vi "displayConfigurableElements.vi"(11 "ConfigurationThisComponent in":refnum<class "ConfigurationTestParameters.lvclass">) -> (3 "ConfigurationThisComponent out":refnum<class "ConfigurationTestParameters.lvclass">)   [LabVIEW 2016, in "ConfigurationTestParameters.lvclass"]
uses:
  ConfigurationTestParameters.lvclass
  Common_Log/Config/Log.ctl
  Typedefs/Device Configuration Tests.ctl
  Typedefs/1-Wire Test.ctl
  Typedefs/Collection Settings.ctl
  Typedefs/TestExecutionOrder.ctl
  Typedefs/TestScenarioTypes.ctl
  Typedefs/Set DAC Tests.ctl
  Typedefs/Set DAC Test.ctl
  Typedefs/Verify DAC Tests.ctl
  Typedefs/DAC Channels.ctl
  Typedefs/Verify DAC Test.ctl
  Typedefs/Verify Voltage Tests.ctl
  Typedefs/Verify Voltage Test.ctl
  Typedefs/Enable Disable.ctl
  Typedefs/Pressure Tests.ctl
  Typedefs/Pressure Test.ctl
  Common_Log/Log.lvlib
  Typedefs/ILCBTTypedefs.lvlib
panel:
  in  "ctrlRefArrayUsrEvnt":refnum<user-event>
  in  "ConfigTab":T1(tab)
  in  "TestDataLog":T2={"Log Directory"=path "", "Log Filename Base"="", "Max records per file"=1000, "Comment"=""} {"Max records per file" min=100 max=1000000}
  in  "TestExecutionOrder":T3
  in  "Collection Settings":T5={"Samples To Average"=1, "Test Delay"=0.01, "Linearity Step"=1024}
  in  "Device Configuration Tests":T6
  in  "Set DAC Tests":T8={"DAC = 0.00A"={"Command Value"=34224}, "DAC = 0.25A"={"Command Value"=42052}, "DAC = 0.5A"={"Command Value"=49879}, "DAC = 0.75A"={"Command Value"=57707}, "DAC = 1.0A"={"Command Value"=65535}, "DAC = -0.25A"={"Command Value"=26396}, "DAC = -0.5A"={"Command Value"=18568}, "DAC = -0.75A"={"Command Value"=10740}, "DAC = -1.0A"={"Command Value"=0}}
  in  "Verify DAC Tests":T10={"DAC A Channels"={"DAQ Channel 1 to Read"="ai5", "DAQ Channel 2 to Read"="ai6", "Resistor Ohms"=0.0}, "DAC B Channels"={"DAQ Channel 1 to Read"="ai7", "DAQ Channel 2 to Read"="ai8", "Resistor Ohms"=0.0}, "DAC = -1.00A"={"Expected Value"=-1.0, "Tolerance"=0.001}, "DAC = -0.75A"={"Expected Value"=-0.75, "Tolerance"=0.00075}, "DAC = -0.50A"={"Expected Value"=-0.5, "Tolerance"=0.0005}, "DAC = -0.25A"={"Expected Value"=-0.25, "Tolerance"=0.00025}, "DAC = 0.00A"={"Expected Value"=0.0, "Tolerance"=0.0001}, "DAC = 0.25A"={"Expected Value"=0.25, "Tolerance"=0.00025}, "DAC = 0.50A"={"Expected Value"=0.5, "Tolerance"=0.0005}, "DAC = 0.75A"={"Expected Value"=0.75, "Tolerance"=0.00075}, "DAC = 1.00A"={"Expected Value"=1.0, "Tolerance"=0.001}} {"DAC = 1.00A"."Tolerance" format="%.6f"; "DAC = 1.00A"."Expected Value" format="%.3f"; "DAC = 0.75A"."Tolerance" format="%.6f"; "DAC = 0.75A"."Expected Value" format="%.3f"; "DAC = 0.50A"."Tolerance" format="%.6f"; "DAC = 0.50A"."Expected Value" format="%.3f"; "DAC = 0.25A"."Tolerance" format="%.6f"; "DAC = 0.25A"."Expected Value" format="%.3f"; "DAC = 0.00A"."Tolerance" format="%.6f"; "DAC = 0.00A"."Expected Value" format="%.3f"; "DAC = -0.25A"."Tolerance" format="%.6f"; "DAC = -0.25A"."Expected Value" format="%.3f"; "DAC = -0.50A"."Tolerance" format="%.6f"; "DAC = -0.50A"."Expected Value" format="%.3f"; "DAC = -0.75A"."Tolerance" format="%.6f"; "DAC = -0.75A"."Expected Value" format="%.3f"; "DAC = -1.00A"."Tolerance" format="%.6f"; "DAC = -1.00A"."Expected Value" format="%.3f"; "DAC B Channels"."Resistor Ohms" format="%.3g"; "DAC A Channels"."Resistor Ohms" format="%.3g"}
  in  "Verify Voltage Tests":T13={"+3.3VD"={"DAQ Channel to Read"="ai0", "Expected Value"=3.3, "Tolerance"=0.0033}, "+5.1V"={"DAQ Channel to Read"="ai1", "Expected Value"=5.1, "Tolerance"=0.0051}, "RELVALV1"={"DAQ Channel to Read"="ai3", "Expected Value"=2.4, "Tolerance"=0.0024}, "RELVALV2"={"DAQ Channel to Read"="ai4", "Expected Value"=2.4, "Tolerance"=0.0024}} {"RELVALV2"."Tolerance" format="%.6f"; "RELVALV2"."Expected Value" format="%.3f"; "RELVALV1"."Tolerance" format="%.6f"; "RELVALV1"."Expected Value" format="%.3f"; "+5.1V"."Tolerance" format="%.6f"; "+5.1V"."Expected Value" format="%.3f"; "+3.3VD"."Tolerance" format="%.6f"; "+3.3VD"."Expected Value" format="%.3f"}
  in  "Enable Disable":T15={"Motor Enable"=1, "Motor Disable"=0, "Current Output Enable"=1, "Current Output Disable"=0, "Power Enable"=0, "Power Disable"=1, "Amplifier Enable"=0, "Amplifier Disable"=1}
  in  "Pressure Tests":T16={"0% Test"={"Command"=0, "Expected"=1933, "Tolerance"=492}, "25% Test"={"Command"=12322, "Expected"=4095, "Tolerance"=492}, "50% Test"={"Command"=26326, "Expected"=6553, "Tolerance"=492}, "75% Test"={"Command"=40329, "Expected"=9010, "Tolerance"=492}, "100% Test"={"Command"=54332, "Expected"=11468, "Tolerance"=492}, "Settling (ms)"=500, "Delay (ms)"=10}
  # "Unique ID Test"
  # "TEDS Status Test"
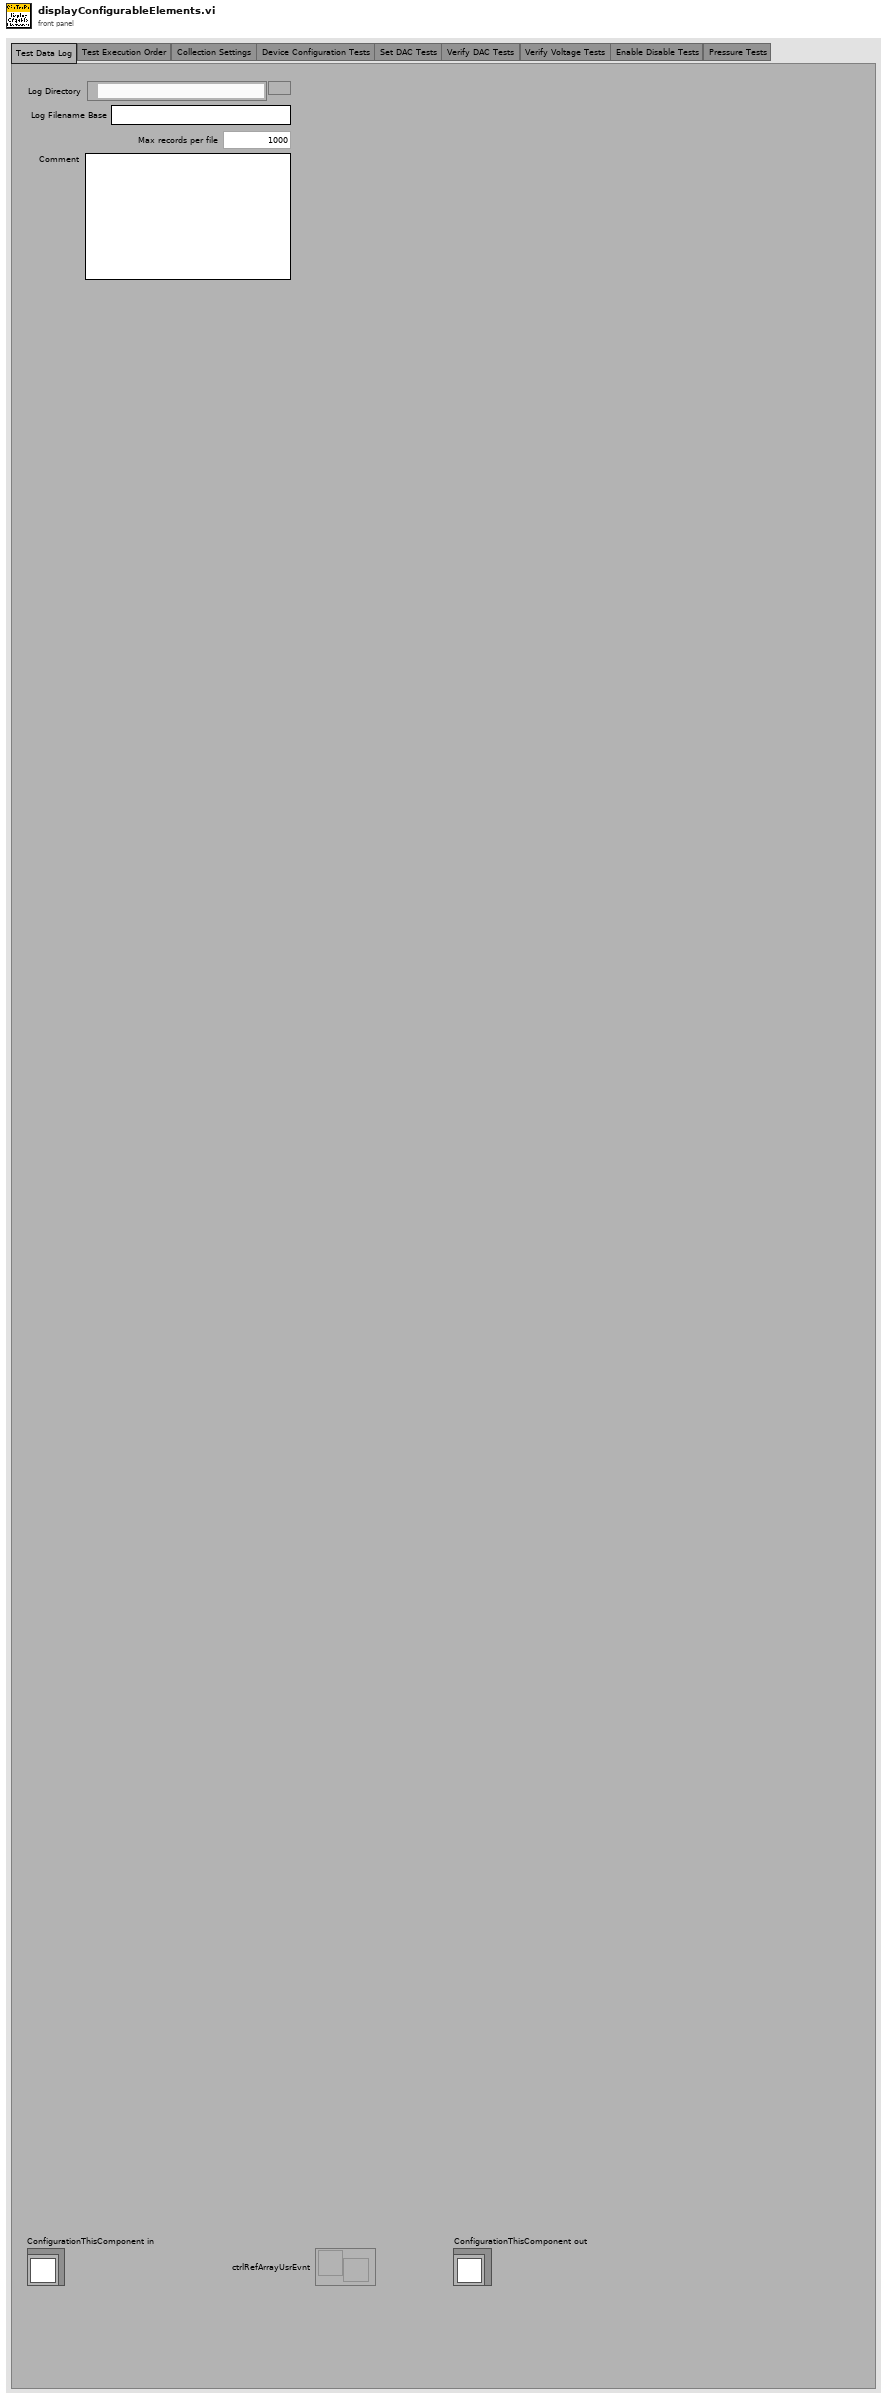
[diagram p1: front panel]
types:
  T1 = enum32{"Test Data Log", "Test Execution Order", "Collection Settings", "Device Configuration Tests", "Set DAC Tests", "Verify DAC Tests", "Verify Voltage Tests", "Enable Disable Tests", "Pressure Tests"}
  T2 = typedef "Log.lvlib/Log.ctl" = cluster{"Log Directory":path, "Log Filename Base":string, "Max records per file":u32, "Comment":string}
  T3 = typedef "ILCBTTypedefs.lvlib/TestExecutionOrder.ctl" = T4[]
  T4 = typedef "ILCBTTypedefs.lvlib/TestScenarioTypes.ctl" = enum16{"+3.3VD", "+5.1V", "+24V", "RELVALV1", "RELVALV2", "Verify DAC_A = -1.00A", "Verify DAC_A = -0.75A", "Verify DAC_A = -0.50A", "Verify DAC_A = -0.25A", "Verify DAC_A = 0.00A", "Verify DAC_A = 0.25A", "Verify DAC_A = 0.50A", "Verify DAC_A = 0.75A", "Verify DAC_A = 1.00A", "Verify DAC_B = -1.00A", "Verify DAC_B = -0.75A", "Verify DAC_B = -0.50A", "Verify DAC_B = -0.25A", "Verify DAC_B = 0.00A", "Verify DAC_B = 0.25A", "Verify DAC_B = 0.50A", "Verify DAC_B = 0.75A", "Verify DAC_B = 1.00A", "Set DAC_A = -1.00A", "Set DAC_A = -0.75A", "Set DAC_A = -0.50A", "Set DAC_A = -0.25A", "Set DAC_A = 0.00A", "Set DAC_A = 0.25A", "Set DAC_A = 0.50A", "Set DAC_A = 0.75A", "Set DAC_A = 1.00A", "Set DAC_B = -1.00A", "Set DAC_B = -0.75A", "Set DAC_B = -0.50A", "Set DAC_B = -0.25A", "Set DAC_B = 0.00A", "Set DAC_B = 0.25A", "Set DAC_B = 0.50A", "Set DAC_B = 0.75A", "Set DAC_B = 1.00A", "Set MTR_PWR = On", "Set MTR_PWR = Off", "Set OUTPUT = On", "Set OUTPUT = Off", "Verify OUTPUT = On", "Verify OUTPUT = Off", "Verify POWER = Ok", "Verify POWER = Fail", "Verify AMP1 = Ok", "Verify AMP1 = Fail", "Verify AMP2 = Ok", "Verify AMP2 = Fail", "P1 0%", "P1 25%", "P1 50%", "P1 75%", "P1 100%", "P2 0%", "P2 25%", "P2 50%", "P2 75%", "P2 100%", "P3 0%", "P3 25%", "P3 50%", "P3 75%", "P3 100%", "P4 0%", "P4 25%", "P4 50%", "P4 75%", "P4 100%", "DCA 1 Linearity", "DCA 2 Linearity"}
  T5 = typedef "ILCBTTypedefs.lvlib/Collection Settings.ctl" = cluster{"Samples To Average":i32, "Test Delay":dbl, "Linearity Step":i32}
  T6 = typedef "ILCBTTypedefs.lvlib/Device Configuration Tests.ctl" = cluster{"TEDS Status Test":T7, "Unique ID Length":u8}
  T7 = typedef "ILCBTTypedefs.lvlib/1-Wire Test.ctl" = cluster{"Expected Value":string}
  T8 = typedef "ILCBTTypedefs.lvlib/Set DAC Tests.ctl" = cluster{"DAC = 0.00A":T9, "DAC = 0.25A":T9, "DAC = 0.5A":T9, "DAC = 0.75A":T9, "DAC = 1.0A":T9, "DAC = -0.25A":T9, "DAC = -0.5A":T9, "DAC = -0.75A":T9, "DAC = -1.0A":T9}
  T9 = typedef "ILCBTTypedefs.lvlib/Set DAC Test.ctl" = cluster{"Command Value":u16}
  T10 = typedef "ILCBTTypedefs.lvlib/Verify DAC Tests.ctl" = cluster{"DAC A Channels":T11, "DAC B Channels":T11, "DAC = -1.00A":T12, "DAC = -0.75A":T12, "DAC = -0.50A":T12, "DAC = -0.25A":T12, "DAC = 0.00A":T12, "DAC = 0.25A":T12, "DAC = 0.50A":T12, "DAC = 0.75A":T12, "DAC = 1.00A":T12}
  T11 = typedef "ILCBTTypedefs.lvlib/DAC Channels.ctl" = cluster{"DAQ Channel 1 to Read":refnum<k21>, "DAQ Channel 2 to Read":refnum<k21>, "Resistor Ohms":dbl}
  T12 = typedef "ILCBTTypedefs.lvlib/Verify DAC Test.ctl" = cluster{"Expected Value":dbl, "Tolerance":dbl}
  T13 = typedef "ILCBTTypedefs.lvlib/Verify Voltage Tests.ctl" = cluster{"+3.3VD":T14, "+5.1V":T14, "RELVALV1":T14, "RELVALV2":T14}
  T14 = typedef "ILCBTTypedefs.lvlib/Verify Voltage Test.ctl" = cluster{"DAQ Channel to Read":refnum<k21>, "Expected Value":dbl, "Tolerance":dbl}
  T15 = typedef "ILCBTTypedefs.lvlib/Enable Disable.ctl" = cluster{"Motor Enable":u16, "Motor Disable":u16, "Current Output Enable":u16, "Current Output Disable":u16, "Power Enable":u16, "Power Disable":u16, "Amplifier Enable":u16, "Amplifier Disable":u16}
  T16 = typedef "ILCBTTypedefs.lvlib/Pressure Tests.ctl" = cluster{"0% Test":T17, "25% Test":T17, "50% Test":T17, "75% Test":T17, "100% Test":T17, "Settling (ms)":u16, "Delay (ms)":u16}
  T17 = typedef "ILCBTTypedefs.lvlib/Pressure Test.ctl" = cluster{"Command":u16, "Expected":u16, "Tolerance":u16}
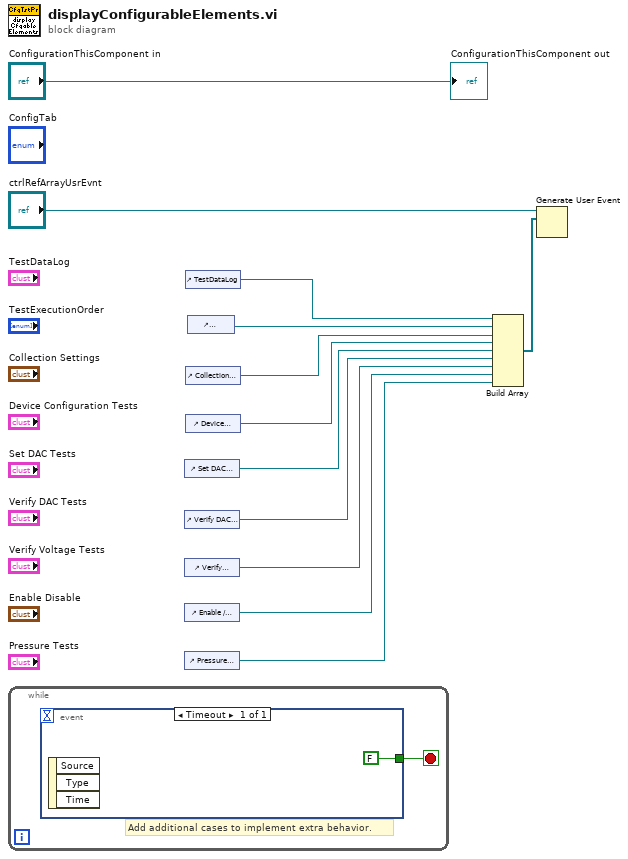
[diagram p0: block diagram]
diagram:
  n1 = while {
    stop <- w13 stop-if-true
    # "Add additional cases to implement extra behavior."
    n2 = event shown="[0] Timeout" {
      selector: _ -> [_]
      dyn-events: _ -> [_]
      timeout: _ -> [_]
      tunnel: [FALSE] -> w13
      event Timeout {
        n3 = event-data() -> ()  [unwired: 1 in, 3 out]
      }
    }
  }
  n4 = control-ref of="Set DAC Tests"() -> (w3:refnum<vi>)
  n5 = control-ref of="Verify DAC Tests"() -> (w4:refnum<vi>)
  n6 = control-ref of="Verify Voltage Tests"() -> (w5:refnum<vi>)
  n7 = control-ref of="Enable / Disable"() -> (w2:refnum<vi>)
  n8 = control-ref of="Pressure Tests"() -> (w1:refnum<vi>)
  n9 = control-ref of="TestDataLog"() -> (w7:refnum<vi>)
  n10 = control-ref of="Collection Settings"() -> (w9:refnum<vi>)
  n11 = control-ref of="Device Configuration Tests"() -> (w6:refnum<vi>)
  n12 = control-ref of="TestExecutionOrder"() -> (w8:refnum<vi>)
  n13 = Build Array(w7, w8, w9, w6, w3, w4, w5, w2, w1) -> (w10:refnum<vi>[])
  n14 = Generate User Event(user event="ctrlRefArrayUsrEvnt", event data cluster=w10) -> ()  [unwired: 2 in, 2 out]
  "ConfigurationThisComponent out" <- "ConfigurationThisComponent in"
